vi "SW_Load_data_for_Conversion_from_TDMS.vi"(8 "error in (no error)":errorcluster, 9 "create index file? (T)":bool, 10 "Data samples to load":i64=-1, 11 "Path to TDMS file":path) -> (0 "error out":errorcluster, 1 "Settings loaded OK":bool, 2 "Data loaded OK":bool, 3 "Loaded data":T1={"Raw coordinates data"=[], "Absolute timestamp"=[], "Relative timestamp"=[], "Coordinates and speed"=[], "Current zone and TTLs"=[], "Zones preference"=[], "Frame OK"=[], "Stimulus presets array"=[], "Acquisition settings cluster out"={"Researcher name"="", "N segments MIDFIELD"=0, "N segments BORDER"=0, "Radius, mm CENTER"=0, "Radius, mm MIDFIELD"=0, "Starting angle MIDFIELD"=0, "Starting angle BORDER"=0, "Cage diameter, mm"=0, "Bridge swap"=FALSE, "Bridge V. offset"=0.0, "Twisted neck"=FALSE, "Offset H."=0.0, "Name prefix"="SavedTrack", "Stop at"=0.0, "\"Stop at\" enabled"=FALSE, "Settings loaded OK"=FALSE}} {"Acquisition settings cluster out"."Stop at" format="%<%H:%M:%S>t"}, 4 "Author's name":string, 5 "Record length, samples":i32, 7 "Time to load, ms":u32)   [LabVIEW 2018]
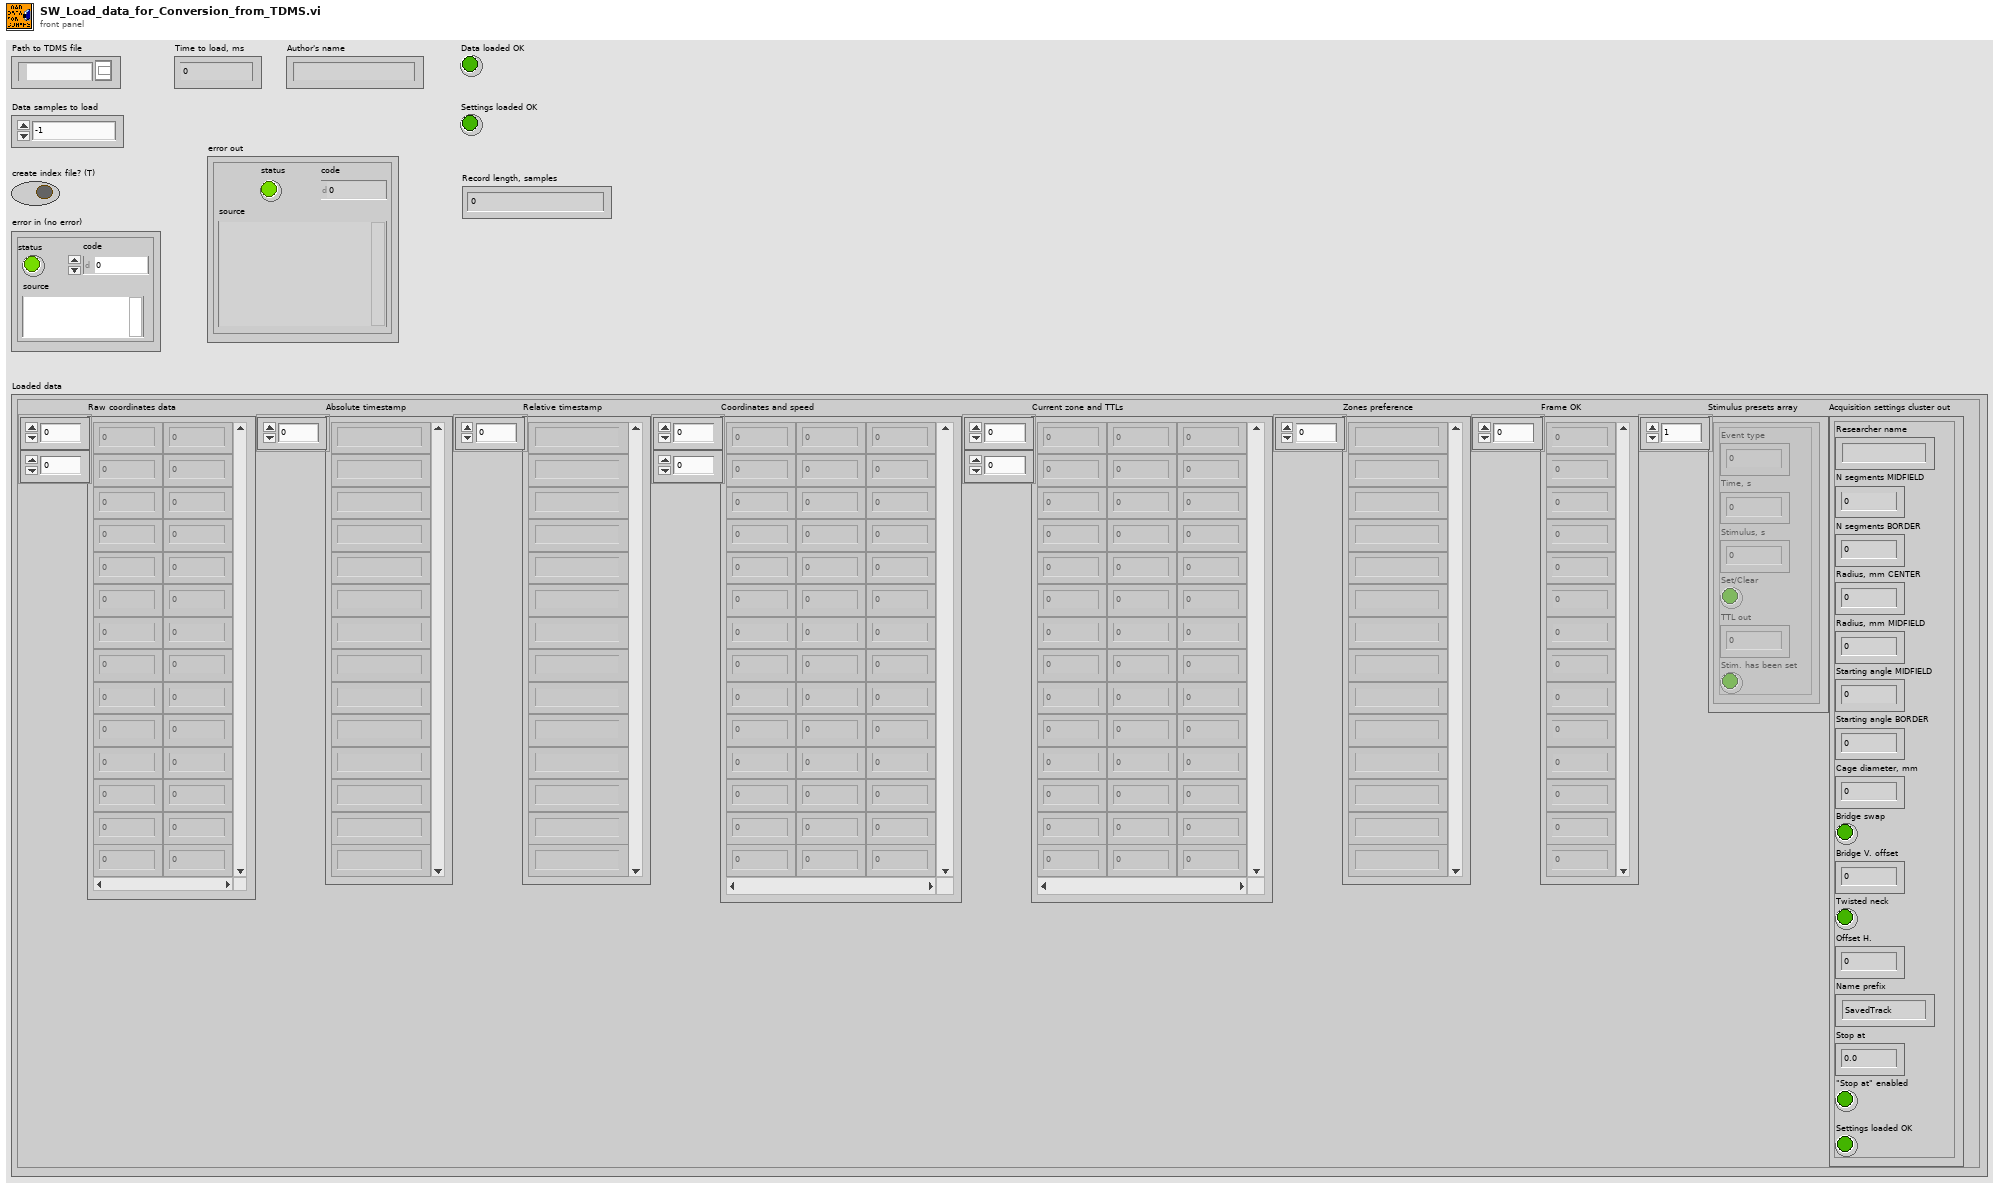
[diagram p1: front panel]
types:
  T1 = cluster{"Raw coordinates data":dbl[][], "Absolute timestamp":string[], "Relative timestamp":string[], "Coordinates and speed":dbl[][], "Current zone and TTLs":u8[][], "Zones preference":string[], "Frame OK":u8[], "Stimulus presets array":cluster{"Event type":u16, "Time, s":sgl, "Stimulus, s":sgl, "Set/Clear":bool, "TTL out":u16, "Stim. has been set":bool}[], "Acquisition settings cluster out":cluster{"Researcher name":string, "N segments MIDFIELD":u8, "N segments BORDER":u8, "Radius, mm CENTER":u16, "Radius, mm MIDFIELD":u16, "Starting angle MIDFIELD":i16, "Starting angle BORDER":i16, "Cage diameter, mm":u16, "Bridge swap":bool, "Bridge V. offset":sgl, "Twisted neck":bool, "Offset H.":sgl, "Name prefix":string, "Stop at":dbl, "\"Stop at\" enabled":bool, "Settings loaded OK":bool}}
  T2 = cluster{"N segments BORDER":u8, "Starting angle BORDER":i16, "N segments MIDFIELD":u8, "Starting angle MIDFIELD":i16, "Radius, mm MIDFIELD":u16, "Amount of central segments":u8, "Radius, mm CENTER":u16, "Bridge swap":bool, "Bridge V. offset":sgl, "Twisted neck":bool, "Offset H.":sgl, "Zones configuration":string[], "IO parameters string":string, "Cage diameter, mm":u16, "Name prefix":string, "Stop at":dbl, "\"Stop at\" enabled":bool}
  T3 = enum16{"big-endian, network order", "native, host order", "little-endian"}
  T4 = enum16{"open", "open or create", "create or replace", "create", "open (read-only)"}
  T5 = cluster{"Event type":u16, "Time, s":sgl, "Stimulus, s":sgl, "Set/Clear":bool, "TTL out":u16, "Stim. has been set":bool}
  T6 = cluster{string, "N segments MIDFIELD":u8, "N segments BORDER":u8, "Radius, mm CENTER":u16, "Radius, mm MIDFIELD":u16, "Starting angle MIDFIELD":i16, "Starting angle BORDER":i16, "Cage diameter, mm":u16, "Bridge swap":bool, "Bridge V. offset":sgl, "Twisted neck":bool, "Offset H.":sgl, "Name prefix":string, "Stop at":dbl, "\"Stop at\" enabled":bool, bool}
  T7 = cluster{dbl[][], string[], string[], dbl[][], u8[][], string[], u8[], cluster{"Event type":u16, "Time, s":sgl, "Stimulus, s":sgl, "Set/Clear":bool, "TTL out":u16, "Stim. has been set":bool}[], cluster{string, "N segments MIDFIELD":u8, "N segments BORDER":u8, "Radius, mm CENTER":u16, "Radius, mm MIDFIELD":u16, "Starting angle MIDFIELD":i16, "Starting angle BORDER":i16, "Cage diameter, mm":u16, "Bridge swap":bool, "Bridge V. offset":sgl, "Twisted neck":bool, "Offset H.":sgl, "Name prefix":string, "Stop at":dbl, "\"Stop at\" enabled":bool, bool}}
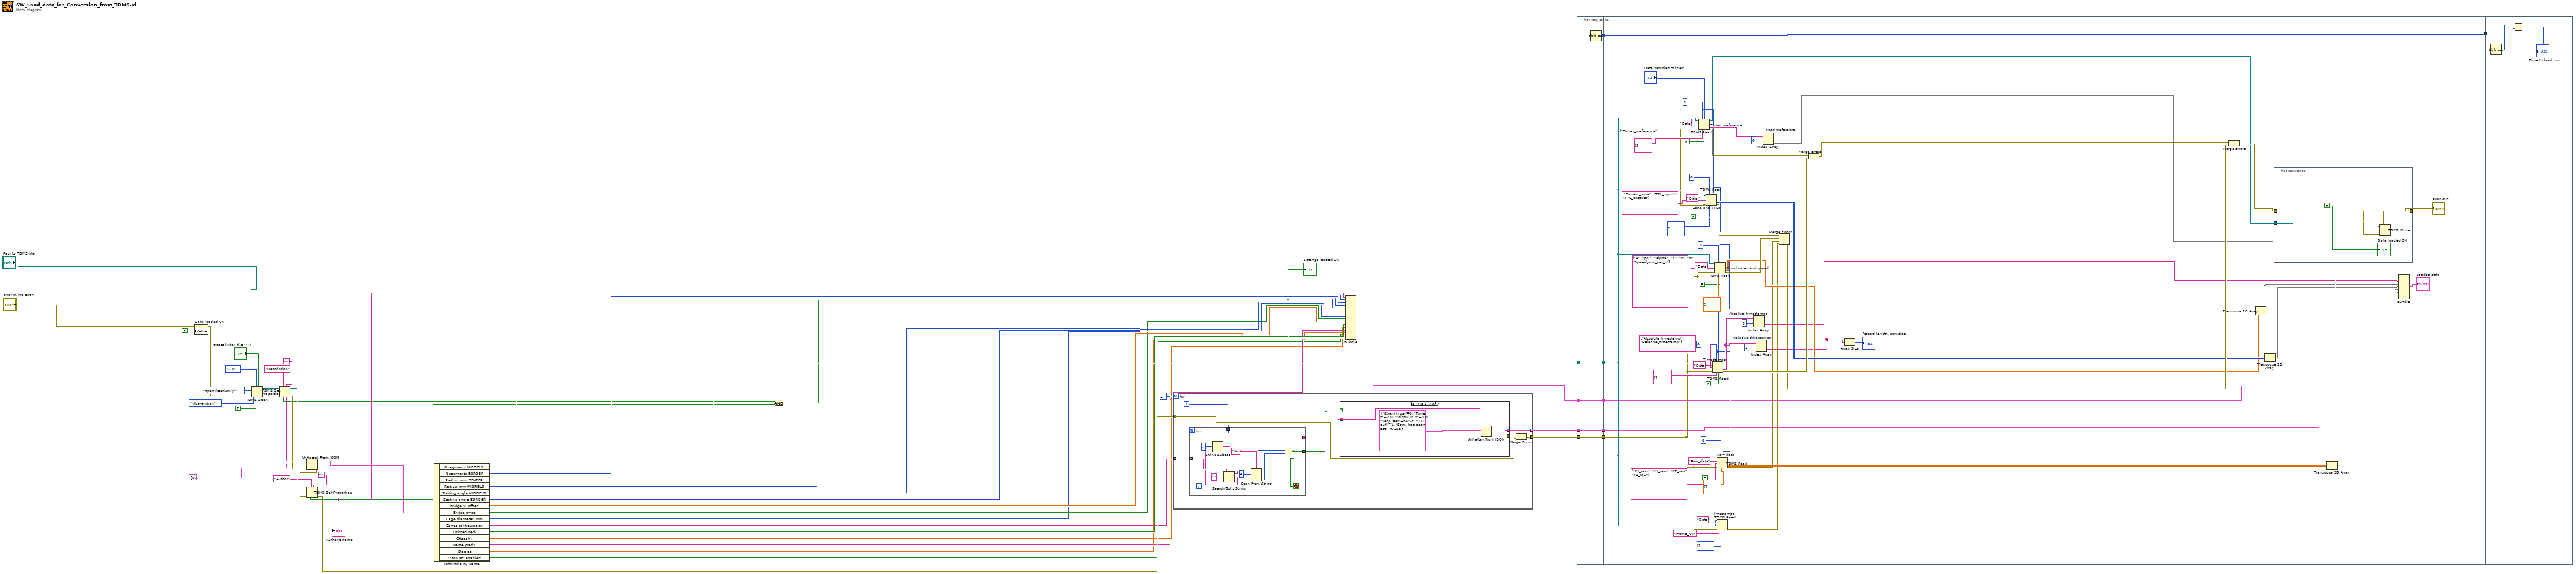
[diagram p0: block diagram]
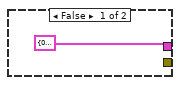
[diagram p2: hidden frame]
diagram:
  n1 = property on="Data loaded OK" class="Bool (strict)"(error in="error in (no error)", "Value"=FALSE ("Data loaded OK")) -> (error out=w17:errorcluster)  [unwired: 1 in, 1 out]
  n2 = TDMS Open(5:"create index file? (T)", 6:TRUE ("disable buffering? (T)"), 7:enum16{"1.0", "2.0"}."2.0" ("file format version (2.0)"), 8:w17, 9:T3."little-endian" ("byte order (2:little-endian)"), 10:T4."open (read-only)" ("operation (0:open)"), 11:"Path to TDMS file") -> (0:w46:errorcluster, 3:w47:refnum<k34>)
  n3 = TDMS Get Properties(5:"", 7:"Description" ("property name"), 8:w46, 11:w47) -> (0:w42:errorcluster, 3:w41:refnum<k34>, 4:w43:string, 6:w26:bool)  [unwired: 2 in, 2 out]
  n4 = Unflatten From JSON(JSON string=w43, type and defaults=T2 {"N segments BORDER"=0, "Starting angle BORDER"=0, "N segments MIDFIELD"=0, "Starting angle MIDFIELD"=0, "Radius, mm MIDFIELD"=0, "Amount of central segments"=0, "Radius, mm CENTER"=0, "Bridge swap"=FALSE, "Bridge V. offset"=0.0, "Twisted neck"=FALSE, "Offset H."=0.0, "Zones configuration"=[], "IO parameters string"="[12,1,1,0,0,0]", "Cage diameter, mm"=180, "Name prefix"="SavedTrack", "Stop at"=0.0, "\"Stop at\" enabled"=FALSE} ("Parameters"), error in (no error)=w42) -> (value=w28:T2, error out=w38:errorcluster)  [unwired: 4 in]
  n5 = TDMS Get Properties(5:"", 7:"Author" ("property name"), 8:w38, 11:w41) -> (0:w24:errorcluster, 3:w21:refnum<k34>, 4:w37:string, 6:w25:bool)  [unwired: 2 in, 2 out]
  "Author's name" <- w37
  n6 = Unbundle By Name(w28) -> ("N segments MIDFIELD"=w36:u8, "N segments BORDER"=w35:u8, "Radius, mm CENTER"=w34:u16, "Radius, mm MIDFIELD"=w33:u16, "Starting angle MIDFIELD"=w32:i16, "Starting angle BORDER"=w31:i16, "Bridge V. offset"=w30:sgl, "Bridge swap"=w29:bool, "Cage diameter, mm"=w27:u16, "Zones configuration"=w23:string[], "Twisted neck"=w6:bool, "Offset H."=w5:sgl, "Name prefix"=w4:string, "Stop at"=w3:dbl, "\"Stop at\" enabled"=w2:bool)
  n7 = And(x=w26, y=w25) -> (x .and. y?=w7:bool)
  "Settings loaded OK" <- w7
  n8 = for {
    N: 14 -> [_]
    tunnel: w24 -> [w57]
    tunnel: [w59] -> w20
    tunnel: [w60] -> w19 mode=indexing
    tunnel: w23 -> [w55]
    i -> [w56]
    n9 = for {
      tunnel: w55 -> [w71] mode=indexing
      tunnel: w56 -> [w65]
      tunnel: [w64] -> w54
      tunnel: [w63] -> w53
      stop <- w64 stop-if-true
      n10 = Search/Split String(string=w71, search string/char (-)=":") -> (substring before match=w69:string, match + rest of string=w62:string)  [unwired: 1 in, 1 out]
      n11 = String Subset(string=w62, offset (0)=2) -> (substring=w63:string)  [unwired: 1 in]
      n12 = Scan From String(format string="%u", input string=w69, initial scan location=u32 4) -> (output 1=w66:u32)  [unwired: 2 in, 3 out]
      n13 = Equal?(x=w65, y=w66) -> (x = y?=w64:bool)
    }
    n14 = case shown="True" w54 {
      tunnel: w53 -> [_ w76]
      tunnel: [T5 {"Event type"=0, "Time, s"=0.0, "Stimulus, s"=0.0, "Set/Clear"=FALSE, "TTL out"=1, "Stim. has been set"=FALSE} ("Cluster of the stimuls settings") w75] -> w60
      tunnel: [_ w74] -> w58
      frame False {
      }
      frame True {
        n15 = Unflatten From JSON(JSON string=w76, type and defaults=T5 {"Event type"=0, "Time, s"=0.0, "Stimulus, s"=0.0, "Set/Clear"=FALSE, "TTL out"=1, "Stim. has been set"=FALSE} ("Cluster of the stimuls settings")) -> (value=w75:T5, error out=w74:errorcluster)  [unwired: 5 in]
      }
    }
    n16 = Merge Errors(w58, w57) -> (w59:errorcluster)
  }
  n17 = Bundle(w37, "N segments MIDFIELD"=w36, "N segments BORDER"=w35, "Radius, mm CENTER"=w34, "Radius, mm MIDFIELD"=w33, "Starting angle MIDFIELD"=w32, "Starting angle BORDER"=w31, "Cage diameter, mm"=w27, "Bridge swap"=w29, "Bridge V. offset"=w30, "Twisted neck"=w6, "Offset H."=w5, "Name prefix"=w4, "Stop at"=w3, "\"Stop at\" enabled"=w2, w7) -> (w9:T6)  [unwired: 1 in]
  n18 = flat-sequence {
    tunnel: w19 -> [w78]
    tunnel: w9 -> [w79]
    tunnel: w20 -> [w80]
    tunnel: w21 -> [w81]
    tunnel: [w81] -> w15
    tunnel: [w80] -> w14
    tunnel: [w79] -> w13
    tunnel: [w78] -> w12
    tunnel: [w77] -> w11
    tunnel: w15 -> [w97]
    tunnel: w14 -> [w96]
    tunnel: w13 -> [w84]
    tunnel: w12 -> [w85]
    tunnel: w11 -> [w108]
    tunnel: [w108] -> w10
    tunnel: w10 -> [w149]
    frame #0 {
      n19 = Tick Count (ms)() -> (millisecond timer value=w77:u32)
    }
    frame #1 {
      n20 = TDMS Read "Zones preference"(0:w97, 1:i64 0 ("offset (0)"), 2:"Data samples to load", 5:"Data" ("group name in"), 7:string[] ["Zones_preference"] ("Columns Names"), 11:w96, 12:string[][] [], 13:FALSE ("return channels in file order? (F)")) -> (4:w113:refnum<k34>, 10:w119:string[][], 15:w127:errorcluster)  [unwired: 3 out]
      n21 = TDMS Read "Zone and TTLs"(0:w97, 1:i64 0 ("offset (0)"), 2:"Data samples to load", 5:"Data" ("group name in"), 7:string[] ["Current_zone", "TTL_inputs", "TTL_outputs"] ("Columns Names"), 11:w96, 12:u8[][] [], 13:FALSE ("return channels in file order? (F)")) -> (10:w116:u8[][], 15:w125:errorcluster)  [unwired: 4 out]
      n22 = TDMS Read "Timestamps"(0:w97, 1:i64 0 ("offset (0)"), 2:"Data samples to load", 5:"Data" ("group name in"), 7:string[] ["Absolute_timestamp", "Relative_timestamp"] ("Columns Names"), 11:w96, 12:string[][] [], 13:FALSE ("return channels in file order? (F)")) -> (10:w121:string[][], 15:w126:errorcluster)  [unwired: 4 out]
      n23 = TDMS Read "Coordinates and speed"(0:w97, 1:i64 0 ("offset (0)"), 2:"Data samples to load", 5:"Data" ("group name in"), 7:string[] ["R", "phi", "alpha", "X", "Y", "w", "Speed_mm_per_s"] ("Columns Names"), 11:w96, 12:dbl[][] [], 13:FALSE ("return channels in file order? (F)")) -> (10:w115:dbl[][], 15:w118:errorcluster)  [unwired: 4 out]
      n24 = TDMS Read "Raw data"(0:w97, 1:i64 0 ("offset (0)"), 2:"Data samples to load", 5:"Raw_data" ("group name in"), 7:string[] ["X1_raw", "Y1_raw", "X2_raw", "Y2_raw"] ("Columns Names"), 11:w96, 12:dbl[][] [], 13:FALSE ("return channels in file order? (F)")) -> (10:w99:dbl[][], 15:w100:errorcluster)  [unwired: 4 out]
      n25 = TDMS Read "Timestamps"(0:w97, 5:"Data" ("group name in"), 7:"Frame_OK" ("channel name(s) in"), 11:w96, 12:u8[] []) -> (10:w86:u8[], 15:w93:errorcluster)  [unwired: 3 in, 4 out]
      n26 = Index Array "Absolute timestamps"(array=w121, index (row)=0) -> (element=w91:string[])  [unwired: 1 in]
      n27 = Index Array "Relative timestamps"(array=w121, index (row)=1) -> (element=w90:string[])  [unwired: 1 in]
      n28 = Index Array "Zones preference"(array=w119, index (row)=0) -> (element=w87:string[])  [unwired: 1 in]
      n29 = Merge Errors(w125, w118, w100, w93) -> (w117:errorcluster)
      n30 = Merge Errors(w127, w126) -> (w82:errorcluster)
      n31 = Array Size(array=w90) -> (size(s)=→"Record length, samples":i32)
      n32 = Merge Errors(w82, w117) -> (w124:errorcluster)
      n33 = Transpose 2D Array(2D array=w115) -> (transposed array=w89:dbl[][])
      n34 = Transpose 2D Array(2D array=w116) -> (transposed array=w88:u8[][])
      n35 = flat-sequence {
        tunnel: [w146] -> w114
        tunnel: w124 -> [w144]
        tunnel: w113 -> [w145]
        frame #0 {
          n36 = TDMS Close(8:w144, 11:w145) -> (0:w146:errorcluster)  [unwired: 1 out]
          "Data loaded OK" <- TRUE ("notification")
        }
      }
      n37 = Transpose 2D Array(2D array=w99) -> (transposed array=w92:dbl[][])
      n38 = Bundle(w92, w91, w90, w89, w88, w87, w86, w85, w84) -> (→"Loaded data":T7)  [unwired: 1 in]
      "error out" <- w114
    }
    frame #2 {
      n39 = Tick Count (ms)() -> (millisecond timer value=w150:u32)
      n40 = Subtract(x=w150, y=w149) -> (x-y=→"Time to load, ms":u32)
    }
  }
